vi "Autonomous Independent.vi"() -> ()   [LabVIEW 2019]
doc: "This VI is called when autonomous begins, and will automatically be terminated when autonomous ends. You can carry out timed or sensor driven robot movement independently without needing to return to the caller."
uses:
  <vilib>/Rock Robotics/WPI/ThirdParty/Phoenix-LabVIEW/Motor Controller/Controls/CTRE_Phoenix_MotorControl_ControlMode.ctl
  <vilib>/Rock Robotics/WPI/Solenoid/WPI_SolenoidValue.ctl
  <vilib>/Rock Robotics/WPI/Utilities/WPI_GetSetVariantRefNum.vi
  <vilib>/Rock Robotics/Network Tables/NT Read String.vi
  <vilib>/Rock Robotics/Network Tables/NT Write Numeric Array.vi
  Robot Global Data.vi
  <vilib>/Rock Robotics/WPI/Solenoid/WPI_SolenoidSetEnum.vi
  <vilib>/Rock Robotics/WPI/RobotDrive/WPI_RobotDriveArcadeDrive_Standard(NoSaturation).vi
panel:
  in  "Output":dbl
  out "Boolean":bool
  out "MVelocity":dbl
  out "WVelocity":dbl
  # "Be sure to right-click and choose Data Operations>>Make Current Value default if you want to save the array values with the VI"
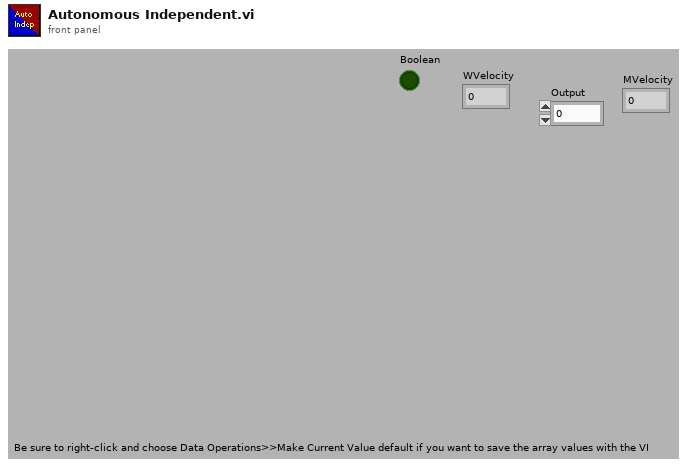
[diagram p1: front panel]
types:
  T1 = typedef "WPI_JoystickDevRef.ctl" = cluster{"Device":T2}
  T2 = typedef "WPI_JoystickDeviceEnum.ctl" = enum16{"USB 0", "USB 1", "USB 2", "USB 3", "USB 4", "USB 5"}
  T3 = typedef "WPI_SolenoidValue.ctl" = enum16{"Off", "On", "Forward", "Reverse"}
  T4 = typedef "WPI_MotorControlDeviceRef.ctl" = cluster{"DeviceStatus":errorcluster, "Type":T5, "PWM":cluster{"PWM Channel":T6, "DeadBand":T7}, "CAN":cluster{"Device Number":u8, "SetOutput VI Ref":variant, "GetOutput VI Ref":variant, "Enable VI Ref":variant, "Disable VI Ref":variant, "Data":variant}, "Invert":bool, "DIO PWM":cluster{"PWM \"Enable\" Channel":T6, "DIOChannel":T8, "PWM Rate":dbl}}
  T5 = typedef "WPI_MotorControlType.ctl" = enum16{"PWM", "CAN", "DIO PWM"}
  T6 = typedef "FPGA_DIOPWMChannel.ctl" = enum8{"PWM 0", "PWM 1", "PWM 2", "PWM 3", "PWM 4", "PWM 5", "PWM 6", "PWM 7", "PWM 8", "PWM 9", "PWM MXP 0", "PWM MXP 1", "PWM MXP 2", "PWM MXP 3", "PWM MXP 4", "PWM MXP 5", "PWM MXP 6", "PWM MXP 7", "PWM MXP 8", "PWM MXP 9", "Invalid"}
  T7 = typedef "WPI_PWMDeadband.ctl" = cluster{"Name":string, "maxPositivePwm":i32, "minPositivePwm":i32, "centerPwm":i32, "maxNegativePwm":i32, "minNegativePwm":i32, "angularRange":u16}
  T8 = typedef "FPGA_DIOChannel.ctl" = enum8{"DIO 0", "DIO 1", "DIO 2", "DIO 3", "DIO 4", "DIO 5", "DIO 6", "DIO 7", "DIO 8", "DIO 9", "DIO MXP 0", "DIO MXP 1", "DIO MXP 2", "DIO MXP 3", "DIO MXP 4", "DIO MXP 5", "DIO MXP 6", "DIO MXP 7", "DIO MXP 8", "DIO MXP 9", "DIO MXP 10", "DIO MXP 11", "DIO MXP 12", "DIO MXP 13", "DIO MXP 14", "DIO MXP 15", "SPI Port CS1", "SPI Port CS2", "SPI Port CS3", "SPI Port MISO", "SPI Port MOSI", "Invalid"}
  T9 = typedef "CTRE_Phoenix_MotorControl_ControlMode.ctl" = u16
  T10 = typedef "WPI_SolenoidDevRef.ctl" = cluster{"DevStatus":errorcluster, "Pneumatics Control Module":u8, "Forward Solenoid Channel":T11, "Reverse Solenoid Channel":T11}
  T11 = typedef "WPI_SolenoidChannel.ctl" = enum8{"Solenoid 0", "Solenoid 1", "Solenoid 2", "Solenoid 3", "Solenoid 4", "Solenoid 5", "Solenoid 6", "Solenoid 7", "Invalid"}
  T12 = typedef "WPI_RobotDriveDevRef.ctl" = cluster{"DevStatus":errorcluster, "Motors[]":T4[], "Square Inputs":bool, "Max Output":dbl}
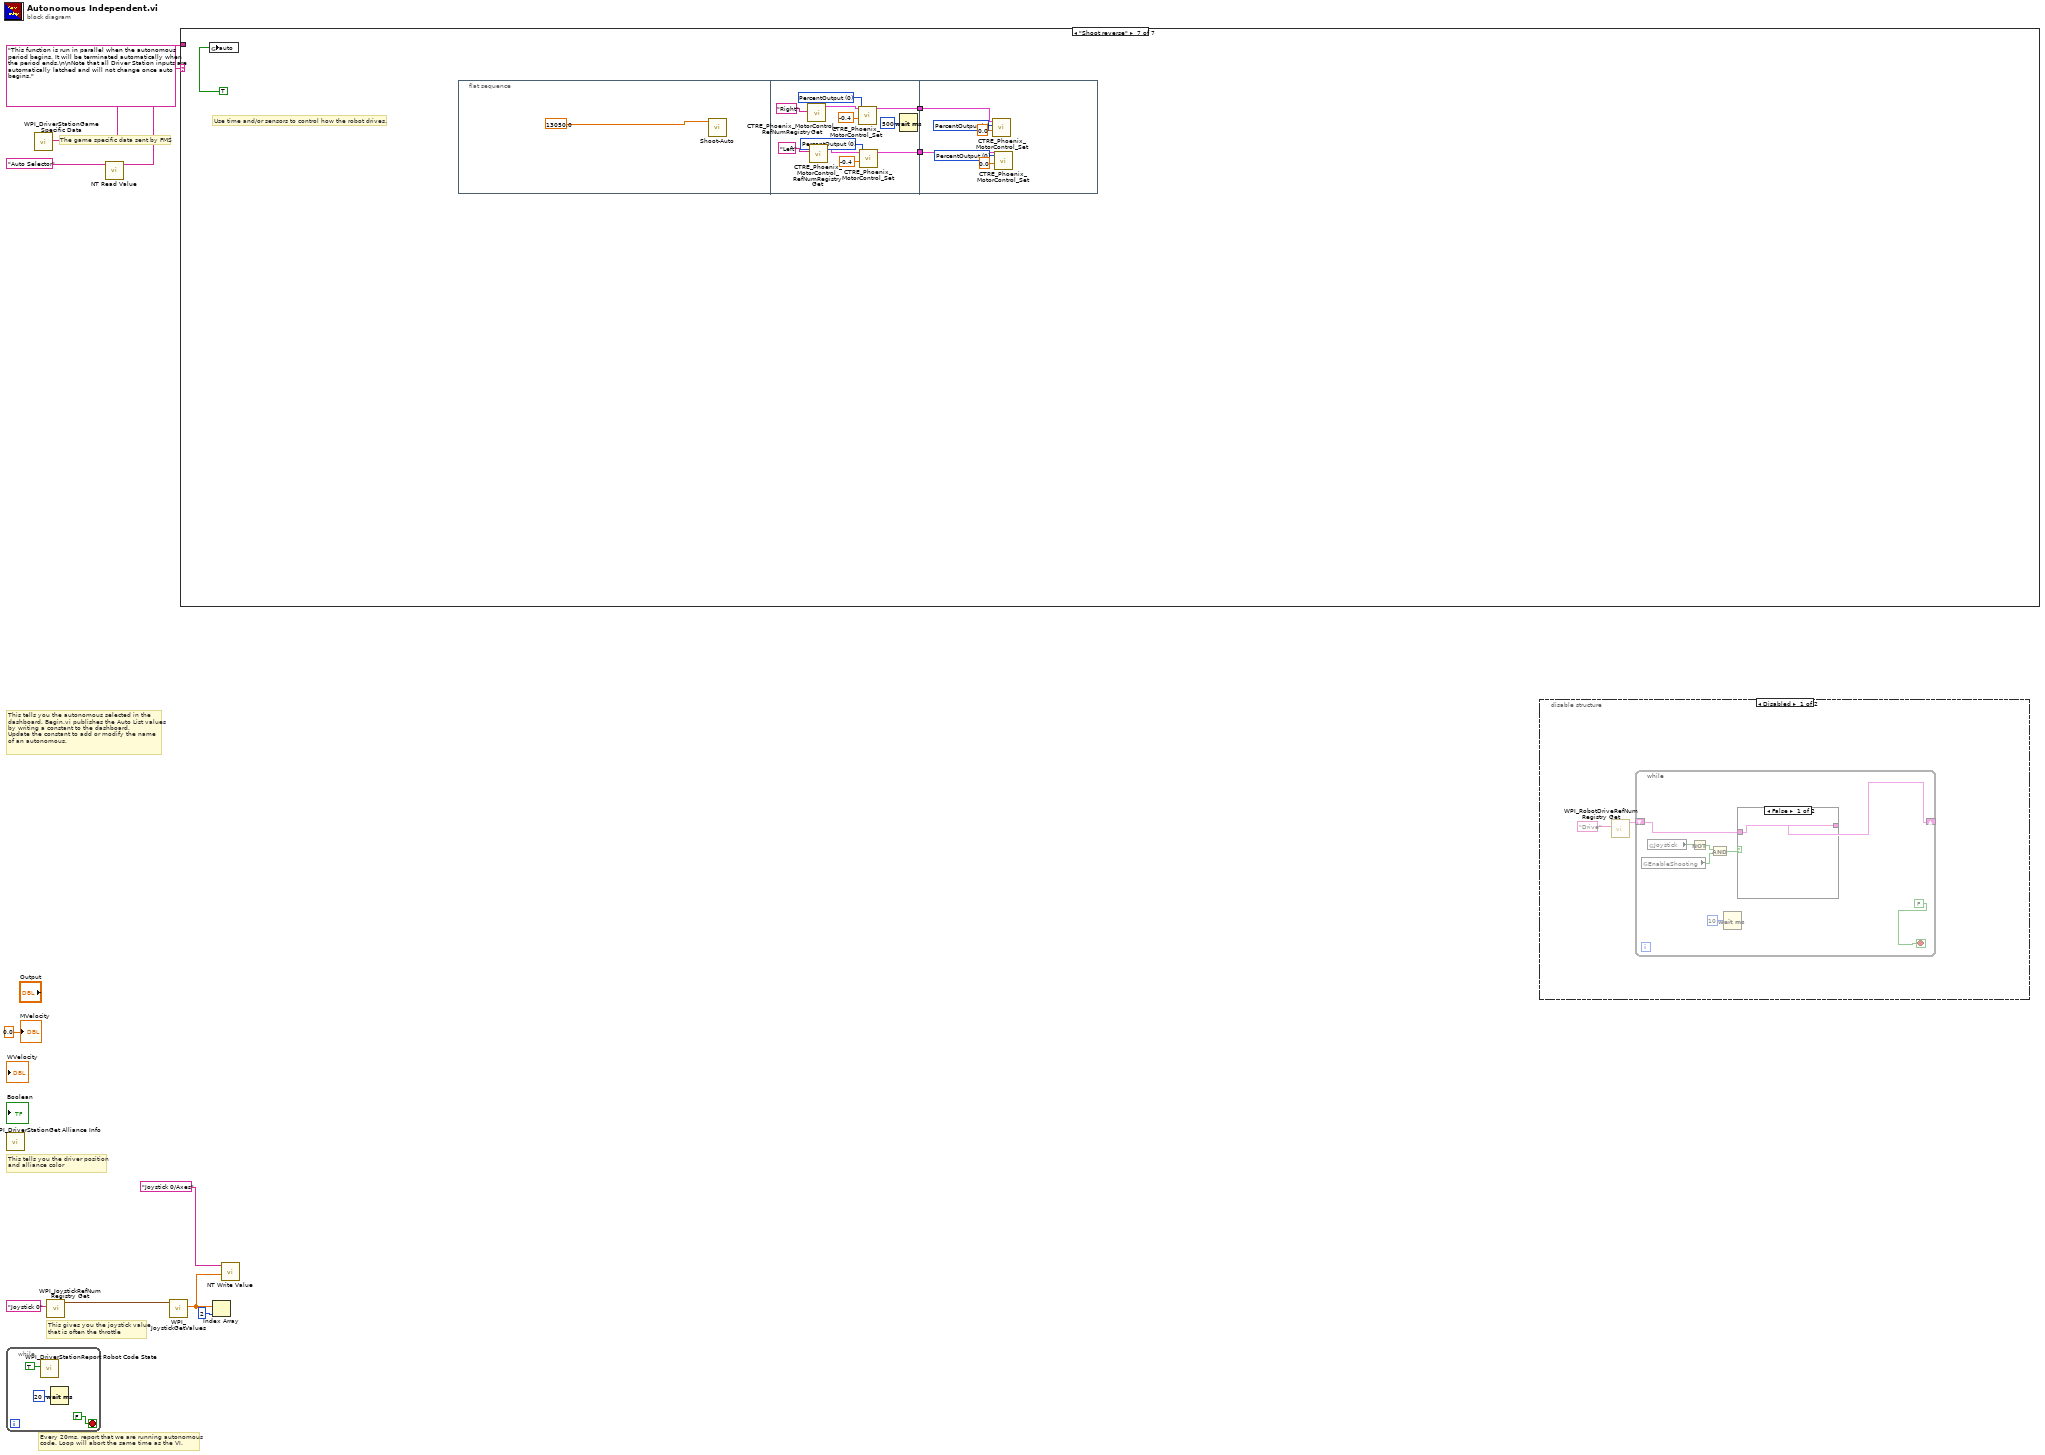
[diagram p0: block diagram]
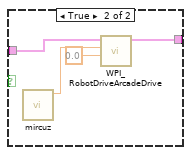
[diagram p2: hidden frame]
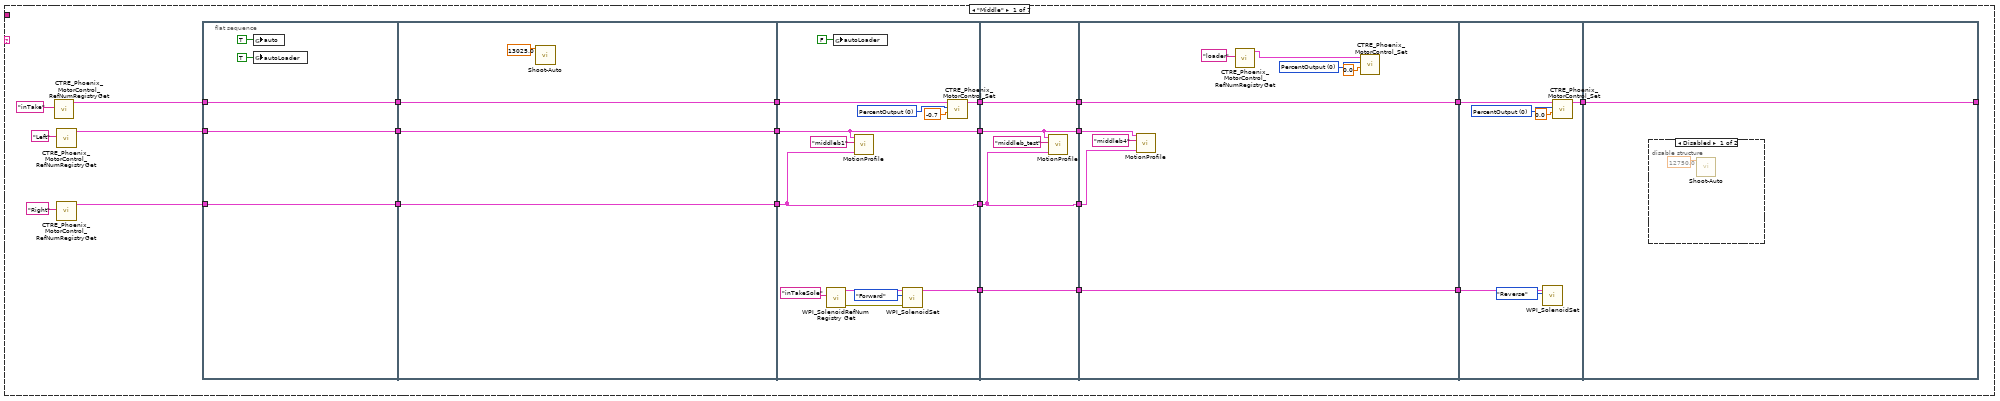
[diagram p4: hidden frame]
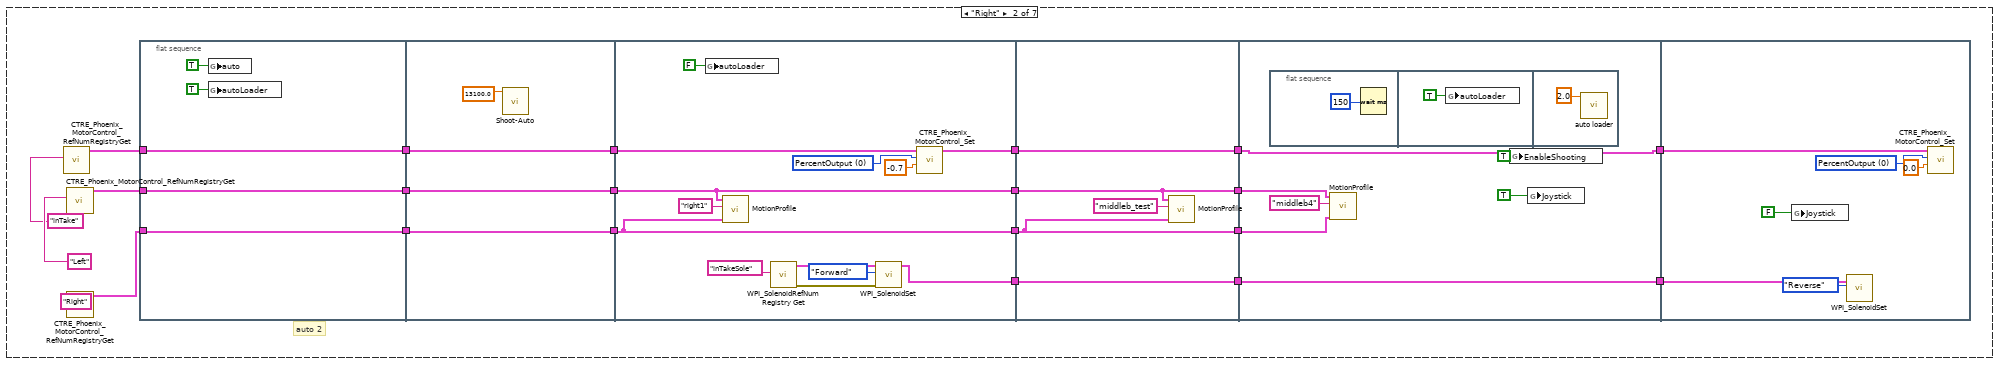
[diagram p6: hidden frame]
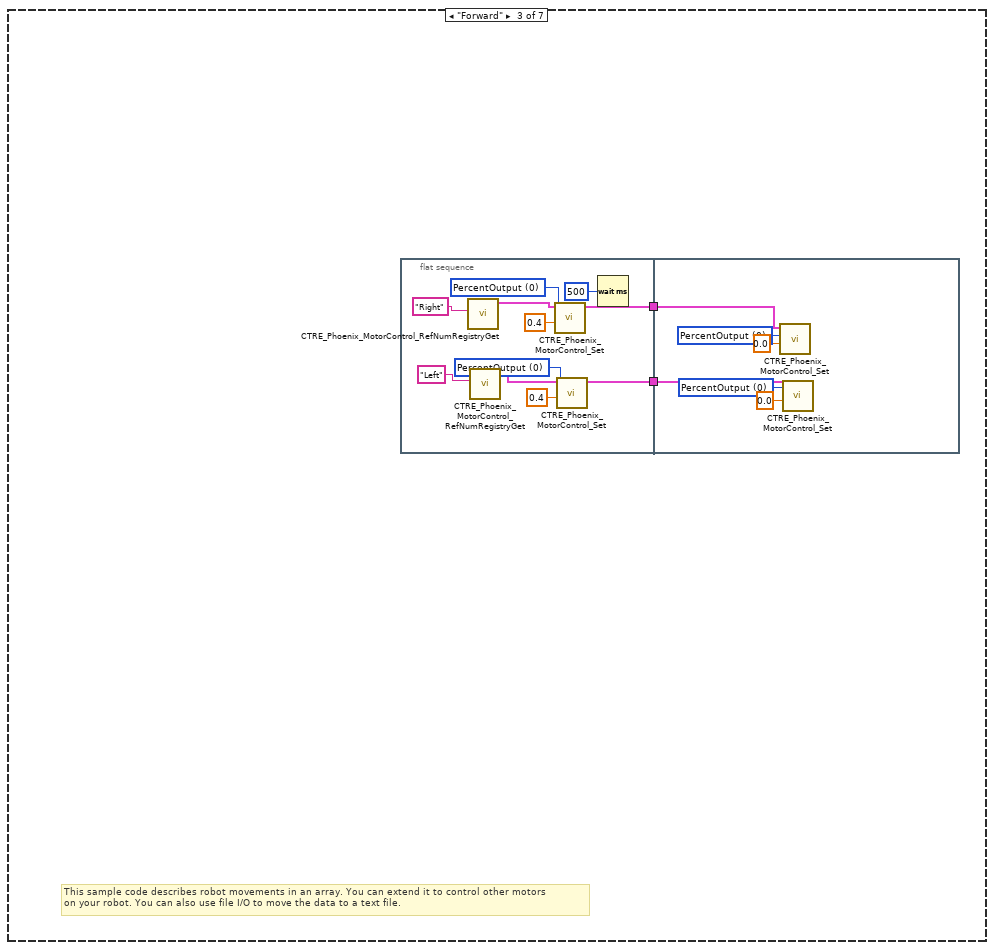
[diagram p7: hidden frame]
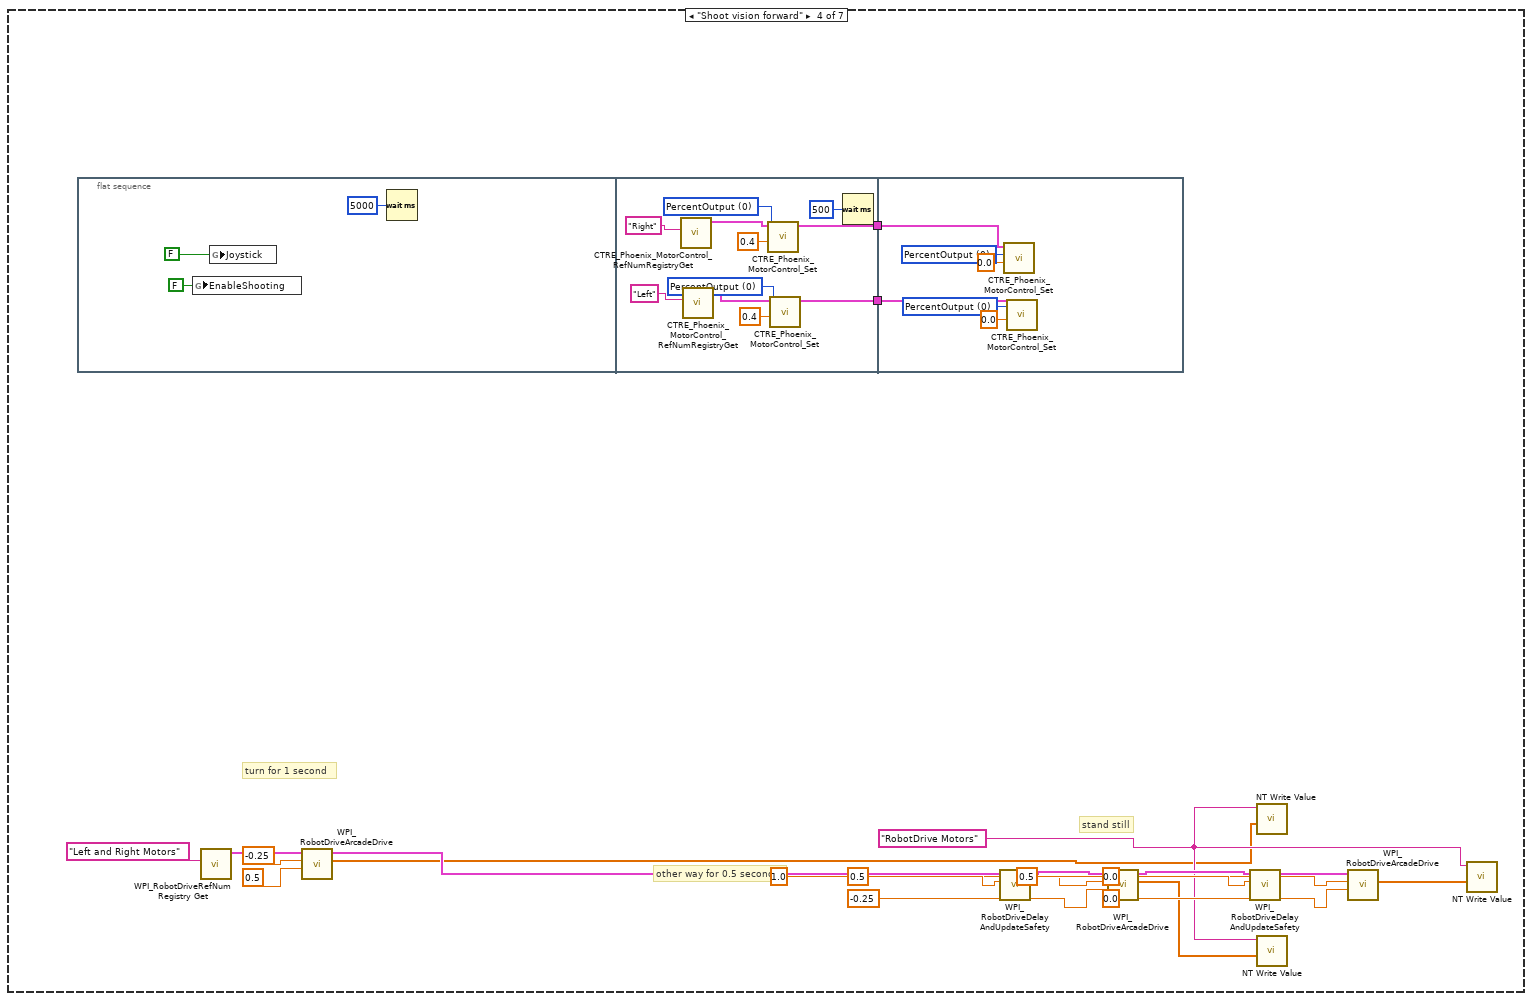
[diagram p8: hidden frame]
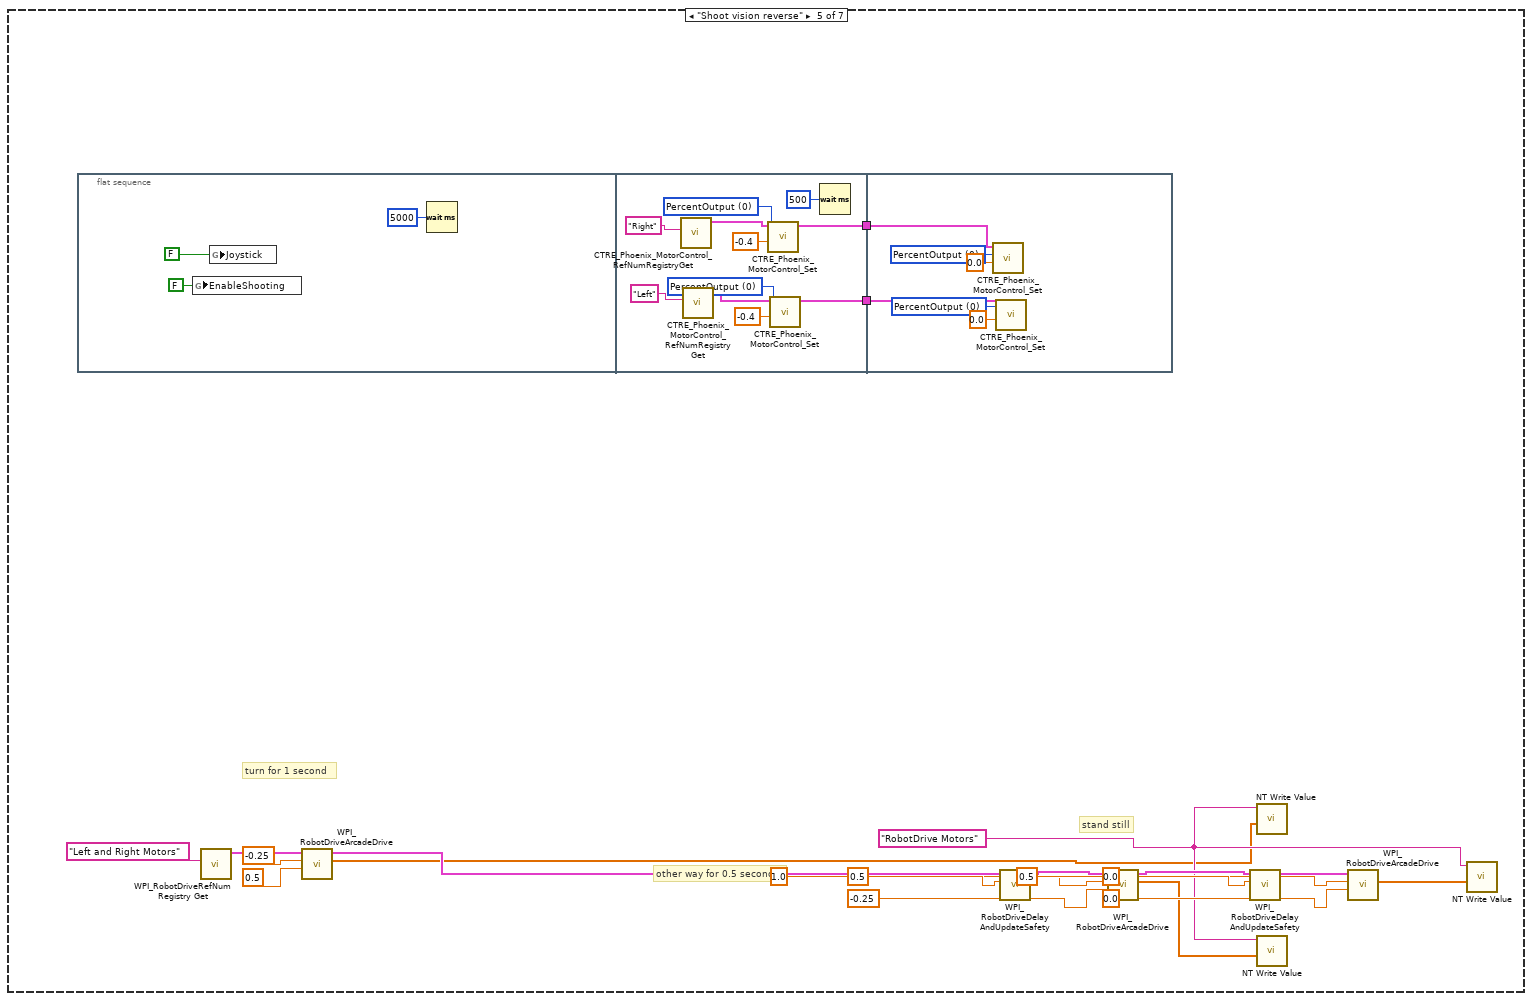
[diagram p9: hidden frame]
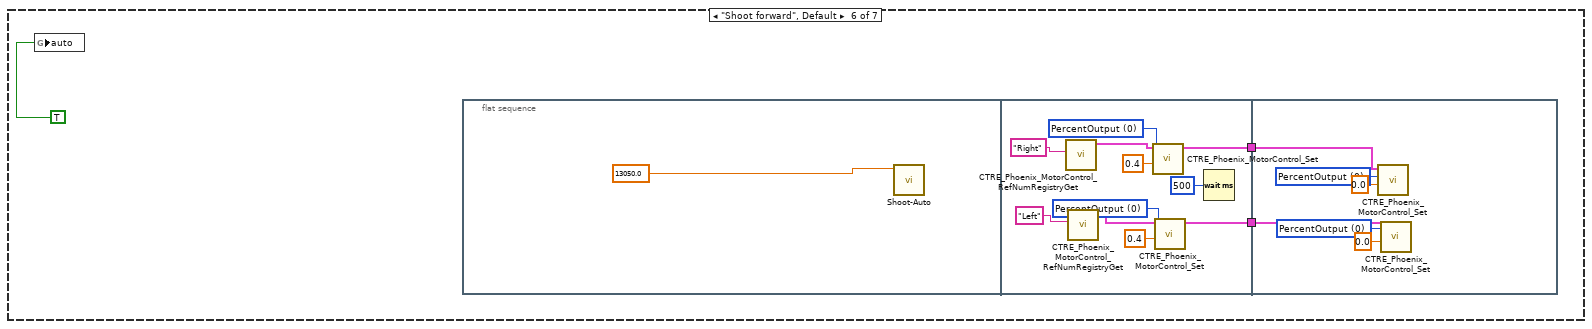
[diagram p10: hidden frame]
diagram:
  (unwired) "This function is run in parallel when the autonomous period begins. It will be terminated automatically when the period ends.\n\nNote that all Driver Station inputs are automatically latched and will not change once auto begins."
  # "The game specific data sent by FMS"
  # "This tells you the autonomous selected in the \ndashboard. Begin.vi publishes the Auto List values\nby writing a constant to the dashboard.\nUpdate the constant to add or modify the name\nof an autonomous."
  # "Every 20ms, report that we are running autonomous\ncode. Loop will abort the same time as the VI."
  # "This gives you the joystick value\nthat is often the throttle"
  # "Use time and/or sensors to control how the robot drives."
  # "This tells you the driver position\nand alliance color"
  n1 = call <vilib>:"WPI_DriverStationGet Alliance Info.vi"() -> ()  [unwired: 12 out]
  n2 = while {
    stop <- FALSE stop-if-true
    n3 = call <vilib>:"WPI_DriverStationReport Robot Code State.vi"("Autonomous"=TRUE) -> ()  [unwired: 10 in, 1 out]
    n4 = Wait (ms)(milliseconds to wait=u32 20) -> ()  [unwired: 1 out]
  }
  n5 = call <vilib>:"WPI_DriverStationGame Specific Data.vi"() -> ("Game Specific Data"=w2:string)  [unwired: 11 in]
  n6 = call <vilib>:"WPI_JoystickRefNum Registry Get.vi"("refnum name"="Joystick 0") -> ("JoystickDevRef"=w8:T1)  [unwired: 1 in, 9 out]
  n7 = call-poly <vilib>:"NT Read Value.vi"("Name"="Auto Selector") -> ("String"=w5:string)  [unwired: 9 in, 1 out]
  n8 = call <vilib>:"WPI_JoystickGetValues.vi"("JoystickDevRef"=w8) -> ("Axes"=w4:dbl[])  [unwired: 6 in, 4 out]
  n9 = case shown="\"Shoot reverse\"" w5 {
    tunnel: w2 -> [_ _ _ _ _ _ _]
    frame "Middle" {
      n10 = call <vilib>:"CTRE_Phoenix_MotorControl_RefNumRegistryGet.vi"("refnum name"="inTake") -> ("PhoenixMotorControlDevRef"=w30:T4)  [unwired: 9 in, 1 out]
      n11 = call <vilib>:"CTRE_Phoenix_MotorControl_RefNumRegistryGet.vi"("refnum name"="Left") -> ("PhoenixMotorControlDevRef"=w32:T4)  [unwired: 9 in, 1 out]
      n12 = call <vilib>:"CTRE_Phoenix_MotorControl_RefNumRegistryGet.vi"("refnum name"="Right") -> ("PhoenixMotorControlDevRef"=w33:T4)  [unwired: 9 in, 1 out]
      n13 = flat-sequence {
        tunnel: w30 -> [w38]
        tunnel: w32 -> [w39]
        tunnel: w33 -> [w40]
        tunnel: [w40] -> w19
        tunnel: [w39] -> w18
        tunnel: [w38] -> w17
        tunnel: [w44] -> w26
        tunnel: [w43] -> w25
        tunnel: [w42] -> w24
        tunnel: w19 -> [w44]
        tunnel: w18 -> [w43]
        tunnel: w17 -> [w42]
        tunnel: [w56] -> w28
        tunnel: [w55] -> w27
        tunnel: [w52] -> w29
        tunnel: w26 -> [w55]
        tunnel: w25 -> [w56]
        tunnel: w24 -> [w51]
        tunnel: [w45] -> w14
        tunnel: w29 -> [w62]
        tunnel: [w62] -> w23
        tunnel: w28 -> [w60]
        tunnel: w27 -> [w59]
        tunnel: [w60] -> w22
        tunnel: [w59] -> w21
        tunnel: [w58] -> w15
        tunnel: w14 -> [w58]
        tunnel: w23 -> [w68]
        tunnel: w22 -> [w70]
        tunnel: w21 -> [w69]
        tunnel: [w68] -> w20
        tunnel: [w67] -> w16
        tunnel: w15 -> [w67]
        tunnel: w20 -> [w75]
        tunnel: w16 -> [w73]
        tunnel: [w74] -> w13
        tunnel: [w78] -> _
        tunnel: w13 -> [w78]
        frame #0 {
          n14 = global write "Robot Global Data.vi" "auto"(TRUE ("auto")) -> ()
          n15 = global write "Robot Global Data.vi" "autoLoader"(TRUE ("auto")) -> ()
        }
        frame #1 {
          n16 = call "Shoot-Auto.vi"("Output"=13025.0) -> ()  [unwired: 11 in]
        }
        frame #2 {
          w53 = T9 0 items=["PercentOutput"=0, "Position"=1, "Velocity"=2, "Current"=3, "Follower"=5, "MotionProfile"=6, "MotionMagic"=7, "MotionProfileArc"=10, "Disabled"=15] ("Control Mode")
          n17 = call <vilib>:"WPI_SolenoidRefNum Registry Get.vi"("refnum name"="inTakeSole") -> ("error out"=w48:errorcluster, "SolenoidDevRef"=w47:T10)  [unwired: 9 in]
          n18 = global write "Robot Global Data.vi" "autoLoader"(FALSE ("auto")) -> ()
          n19 = call "MotionProfile.vi"("Right"=w55, "file name"="middleb1", "Left"=w56) -> ()  [unwired: 9 in]
          n20 = call-poly <vilib>:"WPI_SolenoidSet.vi"("error in (no error)"=w48, "Value"=WPI_SolenoidValue."Forward", "SolenoidDevRef"=w47) -> ("SolenoidDevRef"=w45:T10)  [unwired: 7 in, 1 out]
          n21 = call <vilib>:"CTRE_Phoenix_MotorControl_Set.vi"("Output"=-0.7, "Control Mode"=w53, "PhoenixMotorControlDevRef"=w51) -> ("PhoenixMotorControlDevRef"=w52:T4)  [unwired: 7 in, 1 out]
        }
        frame #3 {
          n22 = call "MotionProfile.vi"("Right"=w59, "file name"="middleb_test", "Left"=w60) -> ()  [unwired: 9 in]
        }
        frame #4 {
          w65 = T9 0 items=["PercentOutput"=0, "Position"=1, "Velocity"=2, "Current"=3, "Follower"=5, "MotionProfile"=6, "MotionMagic"=7, "MotionProfileArc"=10, "Disabled"=15] ("Control Mode")
          n23 = call "MotionProfile.vi"("Right"=w69, "file name"="middleb4", "Left"=w70) -> ()  [unwired: 9 in]
          n24 = call <vilib>:"CTRE_Phoenix_MotorControl_RefNumRegistryGet.vi"("refnum name"="loader") -> ("PhoenixMotorControlDevRef"=w63:T4)  [unwired: 9 in, 1 out]
          n25 = call <vilib>:"CTRE_Phoenix_MotorControl_Set.vi"("Output"=0.0, "Control Mode"=w65, "PhoenixMotorControlDevRef"=w63) -> ()  [unwired: 7 in, 2 out]
        }
        frame #5 {
          w76 = T9 0 items=["PercentOutput"=0, "Position"=1, "Velocity"=2, "Current"=3, "Follower"=5, "MotionProfile"=6, "MotionMagic"=7, "MotionProfileArc"=10, "Disabled"=15] ("Control Mode")
          n26 = call-poly <vilib>:"WPI_SolenoidSet.vi"("Value"=WPI_SolenoidValue."Reverse", "SolenoidDevRef"=w73) -> ()  [unwired: 8 in, 2 out]
          n27 = call <vilib>:"CTRE_Phoenix_MotorControl_Set.vi"("Output"=0.0, "Control Mode"=w76, "PhoenixMotorControlDevRef"=w75) -> ("PhoenixMotorControlDevRef"=w74:T4)  [unwired: 7 in, 1 out]
        }
        frame #6 {
          n28 = disable-structure shown="Disabled" {
            frame Disabled {
              n29 = call "Shoot-Auto.vi"("Output"=12750.0) -> ()  [unwired: 11 in]
            }
            frame Enabled {
            }
          }
        }
      }
    }
    frame "Right" {
      # "auto 2"
      n30 = call <vilib>:"CTRE_Phoenix_MotorControl_RefNumRegistryGet.vi"("refnum name"="inTake") -> ("PhoenixMotorControlDevRef"=w96:T4)  [unwired: 9 in, 1 out]
      n31 = call <vilib>:"CTRE_Phoenix_MotorControl_RefNumRegistryGet.vi"("refnum name"="Left") -> ("PhoenixMotorControlDevRef"=w98:T4)  [unwired: 9 in, 1 out]
      n32 = call <vilib>:"CTRE_Phoenix_MotorControl_RefNumRegistryGet.vi"("refnum name"="Right") -> ("PhoenixMotorControlDevRef"=w97:T4)  [unwired: 9 in, 1 out]
      n33 = flat-sequence {
        tunnel: [w105] -> w88
        tunnel: w98 -> [w105]
        tunnel: w97 -> [w104]
        tunnel: [w104] -> w86
        tunnel: w96 -> [w103]
        tunnel: [w103] -> w84
        tunnel: w88 -> [w110]
        tunnel: [w110] -> w87
        tunnel: w86 -> [w109]
        tunnel: [w109] -> w85
        tunnel: w84 -> [w108]
        tunnel: [w108] -> w83
        tunnel: w87 -> [w118]
        tunnel: w85 -> [w117]
        tunnel: w83 -> [w119]
        tunnel: [w118] -> w95
        tunnel: [w117] -> w92
        tunnel: [w116] -> w91
        tunnel: [w111] -> w80
        tunnel: w95 -> [w127]
        tunnel: [w127] -> w94
        tunnel: [w126] -> w93
        tunnel: w92 -> [w126]
        tunnel: w91 -> [w125]
        tunnel: [w125] -> w90
        tunnel: [w124] -> w81
        tunnel: w80 -> [w124]
        tunnel: w94 -> [w134]
        tunnel: w93 -> [w133]
        tunnel: w90 -> [w132]
        tunnel: [w132] -> w89
        tunnel: [w129] -> w82
        tunnel: w81 -> [w129]
        tunnel: w89 -> [w142]
        tunnel: w82 -> [w139]
        frame #0 {
          n34 = global write "Robot Global Data.vi" "auto"(TRUE ("auto")) -> ()
          n35 = global write "Robot Global Data.vi" "autoLoader"(TRUE ("auto")) -> ()
        }
        frame #1 {
          n36 = call "Shoot-Auto.vi"("Output"=13100.0) -> ()  [unwired: 11 in]
        }
        frame #2 {
          w120 = T9 0 items=["PercentOutput"=0, "Position"=1, "Velocity"=2, "Current"=3, "Follower"=5, "MotionProfile"=6, "MotionMagic"=7, "MotionProfileArc"=10, "Disabled"=15] ("Control Mode")
          n37 = global write "Robot Global Data.vi" "autoLoader"(FALSE ("auto")) -> ()
          n38 = call "MotionProfile.vi"("Right"=w117, "file name"="right1", "Left"=w118) -> ()  [unwired: 9 in]
          n39 = call <vilib>:"WPI_SolenoidRefNum Registry Get.vi"("refnum name"="inTakeSole") -> ("error out"=w114:errorcluster, "SolenoidDevRef"=w113:T10)  [unwired: 9 in]
          n40 = call-poly <vilib>:"WPI_SolenoidSet.vi"("error in (no error)"=w114, "Value"=WPI_SolenoidValue."Forward", "SolenoidDevRef"=w113) -> ("SolenoidDevRef"=w111:T10)  [unwired: 7 in, 1 out]
          n41 = call <vilib>:"CTRE_Phoenix_MotorControl_Set.vi"("Output"=-0.7, "Control Mode"=w120, "PhoenixMotorControlDevRef"=w119) -> ("PhoenixMotorControlDevRef"=w116:T4)  [unwired: 7 in, 1 out]
        }
        frame #3 {
          n42 = call "MotionProfile.vi"("Right"=w126, "file name"="middleb_test", "Left"=w127) -> ()  [unwired: 9 in]
        }
        frame #4 {
          n43 = flat-sequence {
            frame #0 {
              n44 = Wait (ms)(milliseconds to wait=u32 150) -> ()  [unwired: 1 out]
            }
            frame #1 {
              n45 = global write "Robot Global Data.vi" "autoLoader"(TRUE ("auto")) -> ()
            }
            frame #2 {
              n46 = call "auto loader.vi"("balls"=2.0) -> ()  [unwired: 11 in]
            }
          }
          n47 = call "MotionProfile.vi"("Right"=w133, "file name"="middleb4", "Left"=w134) -> ()  [unwired: 9 in]
          n48 = global write "Robot Global Data.vi" "EnableShooting"(TRUE ("auto")) -> ()
          n49 = global write "Robot Global Data.vi" "Joystick"(TRUE ("auto")) -> ()
        }
        frame #5 {
          w143 = T9 0 items=["PercentOutput"=0, "Position"=1, "Velocity"=2, "Current"=3, "Follower"=5, "MotionProfile"=6, "MotionMagic"=7, "MotionProfileArc"=10, "Disabled"=15] ("Control Mode")
          n50 = global write "Robot Global Data.vi" "Joystick"(FALSE ("auto")) -> ()
          n51 = call-poly <vilib>:"WPI_SolenoidSet.vi"("Value"=WPI_SolenoidValue."Reverse", "SolenoidDevRef"=w139) -> ()  [unwired: 8 in, 2 out]
          n52 = call <vilib>:"CTRE_Phoenix_MotorControl_Set.vi"("Output"=0.0, "Control Mode"=w143, "PhoenixMotorControlDevRef"=w142) -> ()  [unwired: 7 in, 2 out]
        }
      }
    }
    frame "Forward" {
      # "This sample code describes robot movements in an array. You can extend it to control other motors\non your robot. You can also use file I/O to move the data to a text file."
      n53 = flat-sequence {
        tunnel: [w149] -> w146
        tunnel: [w148] -> w145
        tunnel: w146 -> [w163]
        tunnel: w145 -> [w162]
        frame #0 {
          w151 = T9 0 items=["PercentOutput"=0, "Position"=1, "Velocity"=2, "Current"=3, "Follower"=5, "MotionProfile"=6, "MotionMagic"=7, "MotionProfileArc"=10, "Disabled"=15] ("Control Mode")
          w153 = T9 0 items=["PercentOutput"=0, "Position"=1, "Velocity"=2, "Current"=3, "Follower"=5, "MotionProfile"=6, "MotionMagic"=7, "MotionProfileArc"=10, "Disabled"=15] ("Control Mode")
          n54 = call <vilib>:"CTRE_Phoenix_MotorControl_RefNumRegistryGet.vi"("refnum name"="Right") -> ("PhoenixMotorControlDevRef"=w154:T4)  [unwired: 9 in, 1 out]
          n55 = call <vilib>:"CTRE_Phoenix_MotorControl_RefNumRegistryGet.vi"("refnum name"="Left") -> ("PhoenixMotorControlDevRef"=w155:T4)  [unwired: 9 in, 1 out]
          n56 = call <vilib>:"CTRE_Phoenix_MotorControl_Set.vi"("Output"=0.4, "Control Mode"=w153, "PhoenixMotorControlDevRef"=w154) -> ("PhoenixMotorControlDevRef"=w148:T4)  [unwired: 7 in, 1 out]
          n57 = call <vilib>:"CTRE_Phoenix_MotorControl_Set.vi"("Output"=0.4, "Control Mode"=w151, "PhoenixMotorControlDevRef"=w155) -> ("PhoenixMotorControlDevRef"=w149:T4)  [unwired: 7 in, 1 out]
          n58 = Wait (ms)(milliseconds to wait=u32 500) -> ()  [unwired: 1 out]
        }
        frame #1 {
          w158 = T9 0 items=["PercentOutput"=0, "Position"=1, "Velocity"=2, "Current"=3, "Follower"=5, "MotionProfile"=6, "MotionMagic"=7, "MotionProfileArc"=10, "Disabled"=15] ("Control Mode")
          w159 = T9 0 items=["PercentOutput"=0, "Position"=1, "Velocity"=2, "Current"=3, "Follower"=5, "MotionProfile"=6, "MotionMagic"=7, "MotionProfileArc"=10, "Disabled"=15] ("Control Mode")
          n59 = call <vilib>:"CTRE_Phoenix_MotorControl_Set.vi"("Output"=0.0, "Control Mode"=w159, "PhoenixMotorControlDevRef"=w162) -> ()  [unwired: 7 in, 2 out]
          n60 = call <vilib>:"CTRE_Phoenix_MotorControl_Set.vi"("Output"=0.0, "Control Mode"=w158, "PhoenixMotorControlDevRef"=w163) -> ()  [unwired: 7 in, 2 out]
        }
      }
    }
    frame "Shoot vision forward" {
      w167 = "RobotDrive Motors" ("Name")
      # "stand still"
      # "other way for 0.5 second"
      # "turn for 1 second"
      n61 = flat-sequence {
        tunnel: [w189] -> w165
        tunnel: [w188] -> w164
        tunnel: w165 -> [w203]
        tunnel: w164 -> [w202]
        frame #0 {
          n62 = global write "Robot Global Data.vi" "EnableShooting"(FALSE ("EnableShooting")) -> ()
          n63 = global write "Robot Global Data.vi" "Joystick"(FALSE ("EnableShooting")) -> ()
          n64 = Wait (ms)(milliseconds to wait=u32 5000) -> ()  [unwired: 1 out]
        }
        frame #1 {
          w191 = T9 0 items=["PercentOutput"=0, "Position"=1, "Velocity"=2, "Current"=3, "Follower"=5, "MotionProfile"=6, "MotionMagic"=7, "MotionProfileArc"=10, "Disabled"=15] ("Control Mode")
          w193 = T9 0 items=["PercentOutput"=0, "Position"=1, "Velocity"=2, "Current"=3, "Follower"=5, "MotionProfile"=6, "MotionMagic"=7, "MotionProfileArc"=10, "Disabled"=15] ("Control Mode")
          n65 = call <vilib>:"CTRE_Phoenix_MotorControl_RefNumRegistryGet.vi"("refnum name"="Right") -> ("PhoenixMotorControlDevRef"=w194:T4)  [unwired: 9 in, 1 out]
          n66 = call <vilib>:"CTRE_Phoenix_MotorControl_RefNumRegistryGet.vi"("refnum name"="Left") -> ("PhoenixMotorControlDevRef"=w195:T4)  [unwired: 9 in, 1 out]
          n67 = call <vilib>:"CTRE_Phoenix_MotorControl_Set.vi"("Output"=0.4, "Control Mode"=w193, "PhoenixMotorControlDevRef"=w194) -> ("PhoenixMotorControlDevRef"=w188:T4)  [unwired: 7 in, 1 out]
          n68 = call <vilib>:"CTRE_Phoenix_MotorControl_Set.vi"("Output"=0.4, "Control Mode"=w191, "PhoenixMotorControlDevRef"=w195) -> ("PhoenixMotorControlDevRef"=w189:T4)  [unwired: 7 in, 1 out]
          n69 = Wait (ms)(milliseconds to wait=u32 500) -> ()  [unwired: 1 out]
        }
        frame #2 {
          w198 = T9 0 items=["PercentOutput"=0, "Position"=1, "Velocity"=2, "Current"=3, "Follower"=5, "MotionProfile"=6, "MotionMagic"=7, "MotionProfileArc"=10, "Disabled"=15] ("Control Mode")
          w199 = T9 0 items=["PercentOutput"=0, "Position"=1, "Velocity"=2, "Current"=3, "Follower"=5, "MotionProfile"=6, "MotionMagic"=7, "MotionProfileArc"=10, "Disabled"=15] ("Control Mode")
          n70 = call <vilib>:"CTRE_Phoenix_MotorControl_Set.vi"("Output"=0.0, "Control Mode"=w199, "PhoenixMotorControlDevRef"=w202) -> ()  [unwired: 7 in, 2 out]
          n71 = call <vilib>:"CTRE_Phoenix_MotorControl_Set.vi"("Output"=0.0, "Control Mode"=w198, "PhoenixMotorControlDevRef"=w203) -> ()  [unwired: 7 in, 2 out]
        }
      }
      n72 = call <vilib>:"WPI_RobotDriveRefNum Registry Get.vi"("refnum name"="Left and Right Motors") -> ("RobotDriveDevRef"=w183:T12)  [unwired: 1 in, 9 out]
      n73 = call-poly <vilib>:"WPI_RobotDriveArcadeDrive.vi"("Y axis value"=0.5 ("X axis value"), "X axis value"=-0.25, "RobotDriveDevRef"=w183) -> ("Motor Values"=w166:dbl[], "RobotDriveDevRef"=w176:T12)  [unwired: 1 in, 6 out]
      n74 = call <vilib>:"WPI_RobotDriveDelayAndUpdateSafety.vi"("Delay (s)"=1.0, "RobotDriveDevRef"=w176) -> ("RobotDriveDevRef 2"=w177:T12)  [unwired: 8 in, 1 out]
      n75 = call-poly <vilib>:"WPI_RobotDriveArcadeDrive.vi"("Y axis value"=-0.25 ("X axis value"), "X axis value"=0.5, "RobotDriveDevRef"=w177) -> ("Motor Values"=w168:dbl[], "RobotDriveDevRef"=w178:T12)  [unwired: 1 in, 6 out]
      n76 = call <vilib>:"WPI_RobotDriveDelayAndUpdateSafety.vi"("Delay (s)"=0.5, "RobotDriveDevRef"=w178) -> ("RobotDriveDevRef 2"=w179:T12)  [unwired: 8 in, 1 out]
      n77 = call-poly <vilib>:"NT Write Value.vi"("Numeric Array"=w166, "Name"=w167) -> ()  [unwired: 9 in, 1 out]
      n78 = call-poly <vilib>:"NT Write Value.vi"("Numeric Array"=w168, "Name"=w167) -> ()  [unwired: 9 in, 1 out]
      n79 = call-poly <vilib>:"WPI_RobotDriveArcadeDrive.vi"("Y axis value"=0.0 ("X axis value"), "X axis value"=0.0, "RobotDriveDevRef"=w179) -> ("Motor Values"=w169:dbl[])  [unwired: 1 in, 7 out]
      n80 = call-poly <vilib>:"NT Write Value.vi"("Numeric Array"=w169, "Name"=w167) -> ()  [unwired: 9 in, 1 out]
    }
    frame "Shoot vision reverse" {
      w207 = "RobotDrive Motors" ("Name")
      # "stand still"
      # "other way for 0.5 second"
      # "turn for 1 second"
      n81 = flat-sequence {
        tunnel: [w229] -> w205
        tunnel: [w228] -> w204
        tunnel: w205 -> [w243]
        tunnel: w204 -> [w242]
        frame #0 {
          n82 = global write "Robot Global Data.vi" "EnableShooting"(FALSE ("EnableShooting")) -> ()
          n83 = global write "Robot Global Data.vi" "Joystick"(FALSE ("EnableShooting")) -> ()
          n84 = Wait (ms)(milliseconds to wait=u32 5000) -> ()  [unwired: 1 out]
        }
        frame #1 {
          w231 = T9 0 items=["PercentOutput"=0, "Position"=1, "Velocity"=2, "Current"=3, "Follower"=5, "MotionProfile"=6, "MotionMagic"=7, "MotionProfileArc"=10, "Disabled"=15] ("Control Mode")
          w233 = T9 0 items=["PercentOutput"=0, "Position"=1, "Velocity"=2, "Current"=3, "Follower"=5, "MotionProfile"=6, "MotionMagic"=7, "MotionProfileArc"=10, "Disabled"=15] ("Control Mode")
          n85 = call <vilib>:"CTRE_Phoenix_MotorControl_RefNumRegistryGet.vi"("refnum name"="Right") -> ("PhoenixMotorControlDevRef"=w234:T4)  [unwired: 9 in, 1 out]
          n86 = call <vilib>:"CTRE_Phoenix_MotorControl_RefNumRegistryGet.vi"("refnum name"="Left") -> ("PhoenixMotorControlDevRef"=w235:T4)  [unwired: 9 in, 1 out]
          n87 = call <vilib>:"CTRE_Phoenix_MotorControl_Set.vi"("Output"=-0.4, "Control Mode"=w233, "PhoenixMotorControlDevRef"=w234) -> ("PhoenixMotorControlDevRef"=w228:T4)  [unwired: 7 in, 1 out]
          n88 = call <vilib>:"CTRE_Phoenix_MotorControl_Set.vi"("Output"=-0.4, "Control Mode"=w231, "PhoenixMotorControlDevRef"=w235) -> ("PhoenixMotorControlDevRef"=w229:T4)  [unwired: 7 in, 1 out]
          n89 = Wait (ms)(milliseconds to wait=u32 500) -> ()  [unwired: 1 out]
        }
        frame #2 {
          w238 = T9 0 items=["PercentOutput"=0, "Position"=1, "Velocity"=2, "Current"=3, "Follower"=5, "MotionProfile"=6, "MotionMagic"=7, "MotionProfileArc"=10, "Disabled"=15] ("Control Mode")
          w239 = T9 0 items=["PercentOutput"=0, "Position"=1, "Velocity"=2, "Current"=3, "Follower"=5, "MotionProfile"=6, "MotionMagic"=7, "MotionProfileArc"=10, "Disabled"=15] ("Control Mode")
          n90 = call <vilib>:"CTRE_Phoenix_MotorControl_Set.vi"("Output"=0.0, "Control Mode"=w239, "PhoenixMotorControlDevRef"=w242) -> ()  [unwired: 7 in, 2 out]
          n91 = call <vilib>:"CTRE_Phoenix_MotorControl_Set.vi"("Output"=0.0, "Control Mode"=w238, "PhoenixMotorControlDevRef"=w243) -> ()  [unwired: 7 in, 2 out]
        }
      }
      n92 = call <vilib>:"WPI_RobotDriveRefNum Registry Get.vi"("refnum name"="Left and Right Motors") -> ("RobotDriveDevRef"=w223:T12)  [unwired: 1 in, 9 out]
      n93 = call-poly <vilib>:"WPI_RobotDriveArcadeDrive.vi"("Y axis value"=0.5 ("X axis value"), "X axis value"=-0.25, "RobotDriveDevRef"=w223) -> ("Motor Values"=w206:dbl[], "RobotDriveDevRef"=w216:T12)  [unwired: 1 in, 6 out]
      n94 = call <vilib>:"WPI_RobotDriveDelayAndUpdateSafety.vi"("Delay (s)"=1.0, "RobotDriveDevRef"=w216) -> ("RobotDriveDevRef 2"=w217:T12)  [unwired: 8 in, 1 out]
      n95 = call-poly <vilib>:"WPI_RobotDriveArcadeDrive.vi"("Y axis value"=-0.25 ("X axis value"), "X axis value"=0.5, "RobotDriveDevRef"=w217) -> ("Motor Values"=w208:dbl[], "RobotDriveDevRef"=w218:T12)  [unwired: 1 in, 6 out]
      n96 = call <vilib>:"WPI_RobotDriveDelayAndUpdateSafety.vi"("Delay (s)"=0.5, "RobotDriveDevRef"=w218) -> ("RobotDriveDevRef 2"=w219:T12)  [unwired: 8 in, 1 out]
      n97 = call-poly <vilib>:"NT Write Value.vi"("Numeric Array"=w206, "Name"=w207) -> ()  [unwired: 9 in, 1 out]
      n98 = call-poly <vilib>:"NT Write Value.vi"("Numeric Array"=w208, "Name"=w207) -> ()  [unwired: 9 in, 1 out]
      n99 = call-poly <vilib>:"WPI_RobotDriveArcadeDrive.vi"("Y axis value"=0.0 ("X axis value"), "X axis value"=0.0, "RobotDriveDevRef"=w219) -> ("Motor Values"=w209:dbl[])  [unwired: 1 in, 7 out]
      n100 = call-poly <vilib>:"NT Write Value.vi"("Numeric Array"=w209, "Name"=w207) -> ()  [unwired: 9 in, 1 out]
    }
    frame "Shoot forward", Default {
      n101 = global write "Robot Global Data.vi" "auto"(TRUE ("auto")) -> ()
      n102 = flat-sequence {
        tunnel: [w250] -> w245
        tunnel: [w249] -> w244
        tunnel: w245 -> [w264]
        tunnel: w244 -> [w263]
        frame #0 {
          n103 = call "Shoot-Auto.vi"("Output"=13050.0) -> ()  [unwired: 11 in]
        }
        frame #1 {
          w252 = T9 0 items=["PercentOutput"=0, "Position"=1, "Velocity"=2, "Current"=3, "Follower"=5, "MotionProfile"=6, "MotionMagic"=7, "MotionProfileArc"=10, "Disabled"=15] ("Control Mode")
          w254 = T9 0 items=["PercentOutput"=0, "Position"=1, "Velocity"=2, "Current"=3, "Follower"=5, "MotionProfile"=6, "MotionMagic"=7, "MotionProfileArc"=10, "Disabled"=15] ("Control Mode")
          n104 = call <vilib>:"CTRE_Phoenix_MotorControl_RefNumRegistryGet.vi"("refnum name"="Right") -> ("PhoenixMotorControlDevRef"=w255:T4)  [unwired: 9 in, 1 out]
          n105 = call <vilib>:"CTRE_Phoenix_MotorControl_RefNumRegistryGet.vi"("refnum name"="Left") -> ("PhoenixMotorControlDevRef"=w256:T4)  [unwired: 9 in, 1 out]
          n106 = call <vilib>:"CTRE_Phoenix_MotorControl_Set.vi"("Output"=0.4, "Control Mode"=w254, "PhoenixMotorControlDevRef"=w255) -> ("PhoenixMotorControlDevRef"=w249:T4)  [unwired: 7 in, 1 out]
          n107 = call <vilib>:"CTRE_Phoenix_MotorControl_Set.vi"("Output"=0.4, "Control Mode"=w252, "PhoenixMotorControlDevRef"=w256) -> ("PhoenixMotorControlDevRef"=w250:T4)  [unwired: 7 in, 1 out]
          n108 = Wait (ms)(milliseconds to wait=u32 500) -> ()  [unwired: 1 out]
        }
        frame #2 {
          w259 = T9 0 items=["PercentOutput"=0, "Position"=1, "Velocity"=2, "Current"=3, "Follower"=5, "MotionProfile"=6, "MotionMagic"=7, "MotionProfileArc"=10, "Disabled"=15] ("Control Mode")
          w260 = T9 0 items=["PercentOutput"=0, "Position"=1, "Velocity"=2, "Current"=3, "Follower"=5, "MotionProfile"=6, "MotionMagic"=7, "MotionProfileArc"=10, "Disabled"=15] ("Control Mode")
          n109 = call <vilib>:"CTRE_Phoenix_MotorControl_Set.vi"("Output"=0.0, "Control Mode"=w260, "PhoenixMotorControlDevRef"=w263) -> ()  [unwired: 7 in, 2 out]
          n110 = call <vilib>:"CTRE_Phoenix_MotorControl_Set.vi"("Output"=0.0, "Control Mode"=w259, "PhoenixMotorControlDevRef"=w264) -> ()  [unwired: 7 in, 2 out]
        }
      }
    }
    frame "Shoot reverse" {
      n111 = global write "Robot Global Data.vi" "auto"(TRUE ("auto")) -> ()
      n112 = flat-sequence {
        tunnel: [w271] -> w266
        tunnel: [w270] -> w265
        tunnel: w266 -> [w285]
        tunnel: w265 -> [w284]
        frame #0 {
          n113 = call "Shoot-Auto.vi"("Output"=13050.0) -> ()  [unwired: 11 in]
        }
        frame #1 {
          w273 = T9 0 items=["PercentOutput"=0, "Position"=1, "Velocity"=2, "Current"=3, "Follower"=5, "MotionProfile"=6, "MotionMagic"=7, "MotionProfileArc"=10, "Disabled"=15] ("Control Mode")
          w275 = T9 0 items=["PercentOutput"=0, "Position"=1, "Velocity"=2, "Current"=3, "Follower"=5, "MotionProfile"=6, "MotionMagic"=7, "MotionProfileArc"=10, "Disabled"=15] ("Control Mode")
          n114 = call <vilib>:"CTRE_Phoenix_MotorControl_RefNumRegistryGet.vi"("refnum name"="Right") -> ("PhoenixMotorControlDevRef"=w276:T4)  [unwired: 9 in, 1 out]
          n115 = call <vilib>:"CTRE_Phoenix_MotorControl_RefNumRegistryGet.vi"("refnum name"="Left") -> ("PhoenixMotorControlDevRef"=w277:T4)  [unwired: 9 in, 1 out]
          n116 = call <vilib>:"CTRE_Phoenix_MotorControl_Set.vi"("Output"=-0.4, "Control Mode"=w275, "PhoenixMotorControlDevRef"=w276) -> ("PhoenixMotorControlDevRef"=w270:T4)  [unwired: 7 in, 1 out]
          n117 = call <vilib>:"CTRE_Phoenix_MotorControl_Set.vi"("Output"=-0.4, "Control Mode"=w273, "PhoenixMotorControlDevRef"=w277) -> ("PhoenixMotorControlDevRef"=w271:T4)  [unwired: 7 in, 1 out]
          n118 = Wait (ms)(milliseconds to wait=u32 500) -> ()  [unwired: 1 out]
        }
        frame #2 {
          w280 = T9 0 items=["PercentOutput"=0, "Position"=1, "Velocity"=2, "Current"=3, "Follower"=5, "MotionProfile"=6, "MotionMagic"=7, "MotionProfileArc"=10, "Disabled"=15] ("Control Mode")
          w281 = T9 0 items=["PercentOutput"=0, "Position"=1, "Velocity"=2, "Current"=3, "Follower"=5, "MotionProfile"=6, "MotionMagic"=7, "MotionProfileArc"=10, "Disabled"=15] ("Control Mode")
          n119 = call <vilib>:"CTRE_Phoenix_MotorControl_Set.vi"("Output"=0.0, "Control Mode"=w281, "PhoenixMotorControlDevRef"=w284) -> ()  [unwired: 7 in, 2 out]
          n120 = call <vilib>:"CTRE_Phoenix_MotorControl_Set.vi"("Output"=0.0, "Control Mode"=w280, "PhoenixMotorControlDevRef"=w285) -> ()  [unwired: 7 in, 2 out]
        }
      }
    }
  }
  n121 = Index Array(array=w4, index=2) -> ()  [unwired: 1 out]
  n122 = call-poly <vilib>:"NT Write Value.vi"("Numeric Array"=w4, "Name"="Joystick 0/Axes") -> ()  [unwired: 9 in, 1 out]
  n123 = disable-structure shown="Disabled" {
    frame Disabled {
      n124 = call <vilib>:"WPI_RobotDriveRefNum Registry Get.vi"("refnum name"="Drive") -> ("RobotDriveDevRef"=w287:T12)  [unwired: 9 in, 1 out]
      n125 = while {
        shift-right: [w293] -> _
        shift-left: w287 -> [w294]
        stop <- FALSE stop-if-true
        n126 = global read "Robot Global Data.vi" "EnableShooting"() -> (w289:bool)
        n127 = global read "Robot Global Data.vi" "Joystick"() -> (w291:bool)
        n128 = Not(x=w291) -> (.not. x?=w290:bool)
        n129 = And(x=w290, y=w289) -> (x .and. y?=w288:bool)
        n130 = Wait (ms)(milliseconds to wait=u32 10) -> ()  [unwired: 1 out]
        n131 = case shown="False" w288 {
          tunnel: w294 -> [w296 w300]
          tunnel: [w296 w299] -> w293
          frame False {
          }
          frame True {
            n132 = call "mircuz.vi"() -> ("x"=w298:dbl)  [unwired: 11 in]
            n133 = call-poly <vilib>:"WPI_RobotDriveArcadeDrive.vi"("Y axis value"=0.0, "X axis value"=w298, "RobotDriveDevRef"=w300) -> ("RobotDriveDevRef"=w299:T12)  [unwired: 6 in, 2 out]
          }
        }
      }
    }
    frame Enabled {
    }
  }
  "MVelocity" <- 0.0 ("MVelocity")
